vi "Scope.vi"(8 "REF_Y":waveform(dbl)[](array[waveform]), 9 "REF_X":waveform(dbl)[](array[waveform]), 10 "AIwfm":waveform(dbl)[](array[waveform]), 11 "AO":waveform(dbl)[](array[waveform])) -> ()   [LabVIEW 2019, in "Instrument.Lockin.lvlib" / "Instrument UI.Lockin.lvclass"]
uses:
  Instrument UI.Lockin.lvclass
panel:
  out "Waveform Graph":waveform(dbl)[](graph)
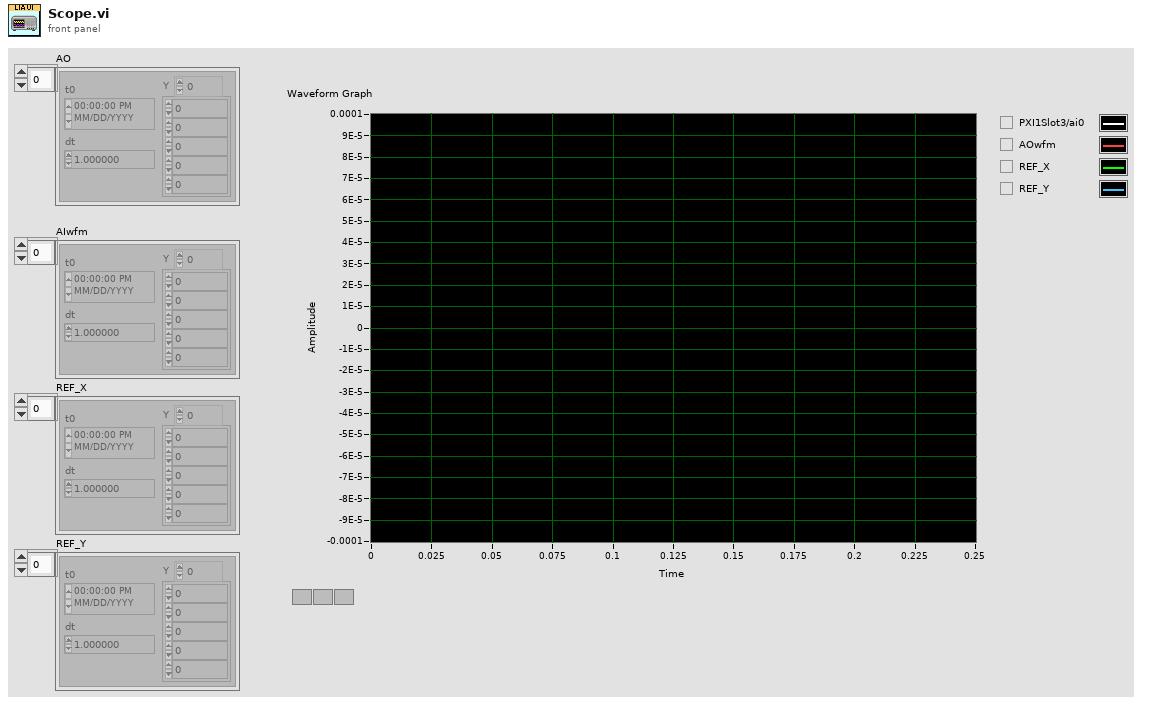
[diagram p1: front panel]
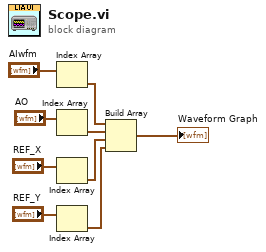
[diagram p0: block diagram]
diagram:
  n1 = Index Array(array="AIwfm") -> (element=w3:waveform(dbl))  [unwired: 1 in]
  n2 = Index Array(array="AO") -> (element=w2:waveform(dbl))  [unwired: 1 in]
  n3 = Index Array(array="REF_X") -> (element=w7:waveform(dbl))  [unwired: 1 in]
  n4 = Index Array(array="REF_Y") -> (element=w4:waveform(dbl))  [unwired: 1 in]
  n5 = Build Array(w3, w2, w7, w4) -> (→"Waveform Graph":waveform(dbl)[])
